vi "Read Array Data.vi"(7 "Section Name":string, 8 "error in (no error)":errorcluster, 10 "Arr Refnum":refnum<vi>, 11 "File Refnum":T1) -> (0 "error out":errorcluster)   [LabVIEW 2013]
uses:
  <vilib>/Utility/config.llb/Config Data RefNum.ctl
  <vilib>/Utility/config.llb/NI_LVConfig.lvlib
panel:
  in  "Sections Regular Expression":string="[0-9A-F]{1,4}(sub[0-9A-f]{1,2}){0,1}"
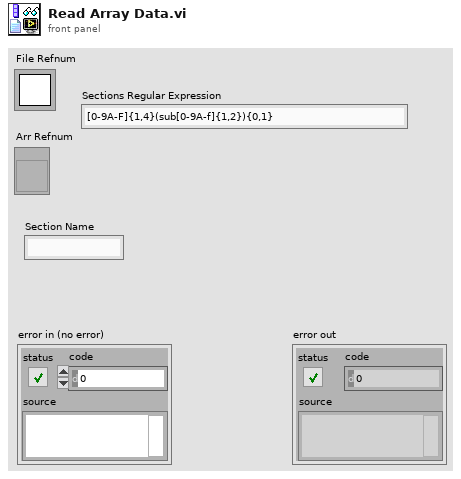
[diagram p1: front panel]
types:
  T1 = typedef "NI_LVConfig.lvlib/Config Data RefNum.ctl" = refnum<k1>
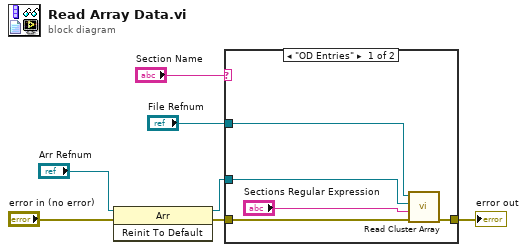
[diagram p0: block diagram]
diagram:
  n1 = invoke class="Arr" method="Reinit To Default"(reference="Arr Refnum", error in="error in (no error)") -> (reference out=w3:refnum<vi>, error out=w1:errorcluster)  [unwired: 1 in, 1 out]
  n2 = case shown="\"OD Entries\"" "Section Name" {
    tunnel: w1 -> [w12 w13]
    tunnel: [w11 w13] -> w6
    tunnel: "File Refnum" -> [w10 _]
    tunnel: w3 -> [w9 _]
    frame "OD Entries" {
      n3 = call "Read Cluster Array.vi"("error in (no error)"=w12, "Regular Expression"="Sections Regular Expression", "Arr Refnum"=w9, "file refnum"=w10) -> ("error out"=w11:errorcluster)  [unwired: 7 in]
    }
    frame "others", Default {
    }
  }
  "error out" <- w6
